vi "Find Tests - When Project Is Not A Refnum - Returns Error.vi"() -> ()   [LabVIEW 2017, in "LVUnit Test Discoverer.Tests.lvlib"]
uses:
  LVUnit Test Discoverer.Tests.lvlib
  LVUnit Test Discoverer/LVUnit Test Discoverer.lvclass
  <vilib>/PNR/Transparent Assertions/Transparent Assertions/Transparent Assertions.lvlib
panel:
  out "error out":errorcluster
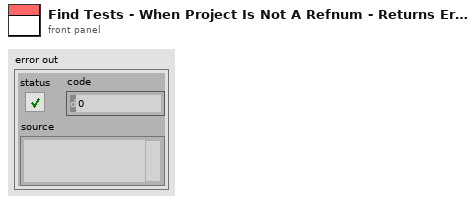
[diagram p1: front panel]
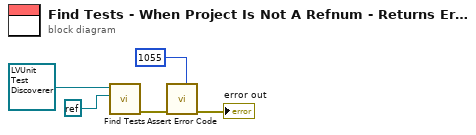
[diagram p0: block diagram]
diagram:
  n1 = call-dynamic "Find Tests.vi"("Project Refnum"=refnum<k0> refnum, "LVUnit Test Discoverer in"=refnum<class "LVUnit Test Discoverer.lvclass"> refnum ("LVUnit Test Discoverer")) -> ("error out"=w3:errorcluster)  [unwired: 7 in, 2 out]
  n2 = call <vilib>:"Assert Error Code.vi"("Expected"=1055, "error in (no error)"=w3) -> ("error out"=→"error out":errorcluster)  [unwired: 9 in]
